vi "Close Comm.vi"(8 "error in (no error)":errorcluster, 11 "AISAS Mech":refnum<class "AISAS Mech.lvclass">) -> (0 "error out":errorcluster)   [LabVIEW 2014, in "AISAS Mech.lvclass"]
uses:
  AISAS Mech.lvclass
  AISAS Mech.lvclass/AISAS Mech.ctl
  motor/AISAS motor.lvclass/AISAS motor.ctl
  motor/AISAS motor.lvclass
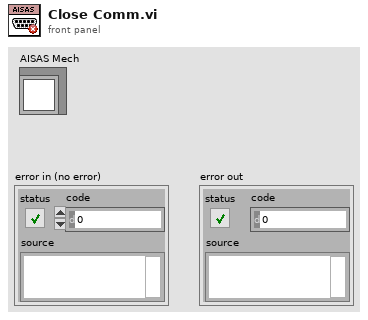
[diagram p1: front panel]
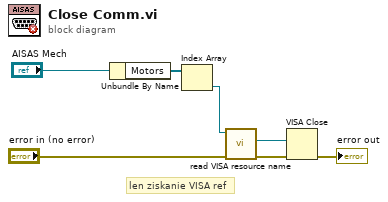
[diagram p0: block diagram]
diagram:
  # "len ziskanie VISA ref"
  n1 = Unbundle By Name("AISAS Mech") -> ("Motors"=w5:refnum<class "AISAS motor.lvclass">[])
  n2 = Index Array(array=w5) -> (element=w4:refnum<class "AISAS motor.lvclass">)  [unwired: 1 in]
  n3 = call "read VISA resource name.vi"("error in (no error)"="error in (no error)", "AISAS motor in"=w4) -> ("error out"=w2:errorcluster, "VISA resource name"=w1:refnum<visa-resource-name>)  [unwired: 7 in, 1 out]
  n4 = VISA Close(VISA resource name=w1, error in (no error)=w2) -> (error out=→"error out":errorcluster)
